vi "Reorder Coefficients.vi"(0 "coefficients":dbl[](array[numeric]), 7 "num coefficients":i32=16, 9 "spc":i32=16) -> (4 "reordered coefficients":dbl[](array[numeric]))   [LabVIEW 2019]
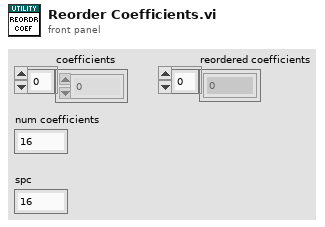
[diagram p1: front panel]
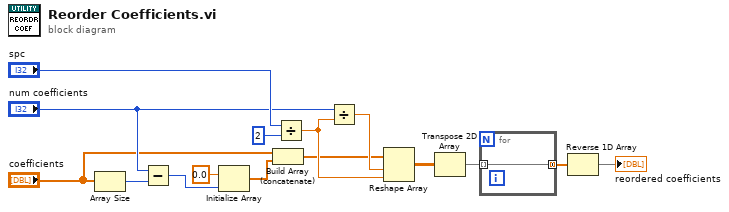
[diagram p0: block diagram]
diagram:
  n1 = Array Size(array="coefficients") -> (size(s)=w7:i32)
  n2 = Subtract(x="num coefficients", y=w7) -> (x-y=w6:i32)
  n3 = Initialize Array(0.0 ("element"), w6) -> (w4:dbl[])
  n4 = Build Array (concatenate)("coefficients", w4) -> (w1:dbl[])
  n5 = Divide(x="spc", y=2) -> (x/y=w14:dbl)
  n6 = Divide(x="num coefficients", y=w14) -> (x/y=w13:dbl)
  n7 = Reshape Array(w1, w13, w14) -> (w12:dbl[][])
  n8 = Transpose 2D Array(2D array=w12) -> (transposed array=w11:dbl[][])
  n9 = for {
    tunnel: [w16] -> w10 mode=concatenating
    tunnel: w11 -> [w16] mode=indexing
  }
  n10 = Reverse 1D Array(array=w10) -> (reversed array=→"reordered coefficients":dbl[])
